vi "Define_KNRm.vi"() -> (0 "error out":errorcluster, 3 "KNR out":T1)   [LabVIEW 2013]
uses:
  <userlib>/KNR OS 3.0 LabVIEW Toolkit/Type Definition/KNR3 Reference.ctl
  <userlib>/_FPGA Interface Advanced Tools/FPGA Interface Base/FPGA Interface Base.lvclass
  <userlib>/KNR OS 3.0 LabVIEW Toolkit/Type Definition/Resource.ctl
  <userlib>/KNR OS 3.0 LabVIEW Toolkit/Type Definition/DC Motor Port.ctl
  <userlib>/KNR OS 3.0 LabVIEW Toolkit/Type Definition/RC Servo Port.ctl
  Global_KNRm.vi
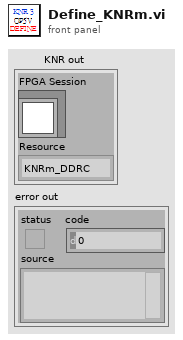
[diagram p1: front panel]
types:
  T1 = typedef "KNR3 Reference.ctl" = cluster{"FPGA Session":refnum<class "FPGA Interface Base.lvclass">, "Resource":T2}
  T2 = typedef "Resource.ctl" = enum16{"KNRm_DDRC", "KNRm_DDDD", "KNRm_DDDR", "KNRm_DDDC", "KNR"}
  T3 = typedef "DC Motor Port.ctl" = u16
  T4 = typedef "RC Servo Port.ctl" = u16
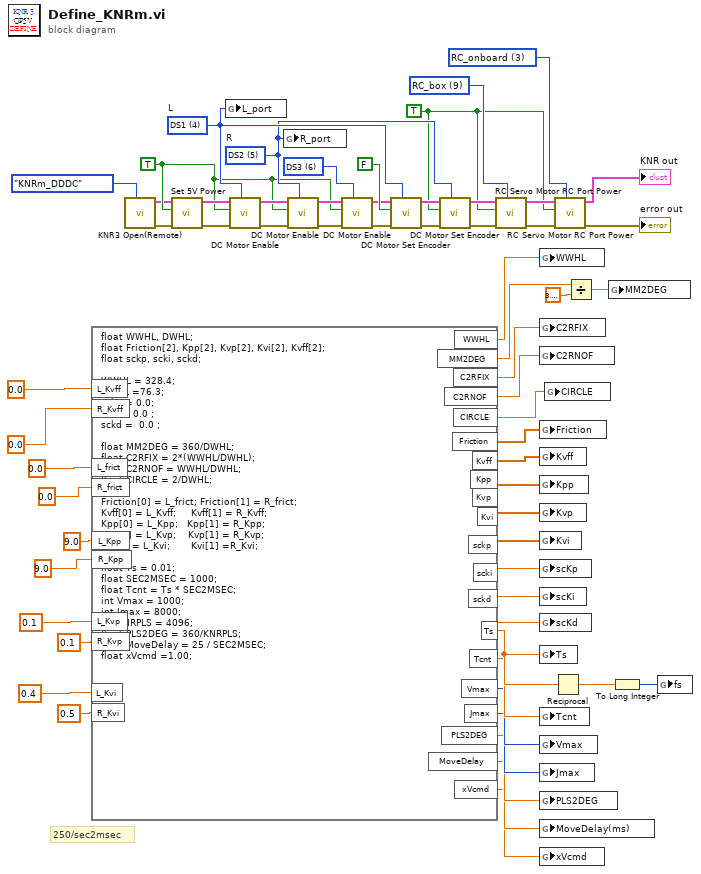
[diagram p0: block diagram]
diagram:
  w23 = T3 6 items=["DS1"=4, "DS2"=5, "DS3"=6, "DS4"=7] ("Port (DS1)")
  w28 = T4 3 items=["RC_onboard"=3, "RC_box"=9] ("Port (RC_onboard)")
  w32 = T4 9 items=["RC_onboard"=3, "RC_box"=9] ("Port (RC_onboard)")
  w56 = T3 5 items=["DS1"=4, "DS2"=5, "DS3"=6, "DS4"=7]  # R
  w57 = T3 4 items=["DS1"=4, "DS2"=5, "DS3"=6, "DS4"=7]  # L
  w29 = TRUE ("Reverse?(F)")
  w15 = TRUE ("Enable Motor(F)")
  # "250/sec2msec"
  n1 = formula code="float WWHL, DWHL;\nfloat Friction[2], Kpp[2], Kvp[2], Kvi[2], Kvff[2];\nfloat sckp, scki, sckd;\n\nWWHL = 328.4;\nDWHL =76.3;\nsckp = 0.0;\nscki = 0.0 ;\nsckd =  0.0 ;\n\nfloat MM2DEG = 360/DWHL;\nfloat C2RFIX = 2*(WWHL/DWHL);\nfloat C2RNOF = WWHL/DWHL;\nfloat CIRCLE = 2/DWHL;\n\nFriction[0] = L_frict; Friction[1] = R_frict;\nKvff[0] = L_Kvff;     Kvff[1] = R_Kvff;\nKpp[0] = L_Kpp;   Kpp[1] = R_Kpp;\nKvp[0] = L_Kvp;    Kvp[1] = R_Kvp;\nKvi[0] = L_Kvi;       Kvi[1] =R_Kvi;\n\nfloat Ts = 0.01;\nfloat SEC2MSEC = 1000;\nfloat Tcnt = Ts * SEC2MSEC;\nint Vmax = 1000;\nint Jmax = 8000;\nint KNRPLS = 4096;\nfloat PLS2DEG = 360/KNRPLS;\nfloat MoveDelay = 25 / SEC2MSEC;\nfloat xVcmd =1.00;"("L_Kvff"=0.0 ("input variable"), "R_Kvff"=0.0 ("input variable"), "L_frict"=0.0 ("input variable"), "R_frict"=0.0 ("input variable"), "L_Kpp"=9.0 ("input variable"), "R_Kpp"=9.0 ("input variable"), "L_Kvp"=0.1 ("input variable"), "R_Kvp"=0.1 ("input variable"), "L_Kvi"=0.4 ("input variable"), "R_Kvi"=0.5 ("input variable")) -> ("MM2DEG"=w20:dbl, "C2RFIX"=w52:dbl, "C2RNOF"=w51:dbl, "Friction"=w50:dbl[], "Kvff"=w49:dbl[], "Kpp"=w48:dbl[], "Kvp"=w47:dbl[], "Kvi"=w46:dbl[], "sckp"=w45:dbl, "scki"=w44:dbl, "sckd"=w43:dbl, "Ts"=w40:dbl, "Tcnt"=w39:dbl, "Vmax"=w38:i32, "Jmax"=w37:i32, "PLS2DEG"=w36:dbl, "WWHL"=w22:dbl, "MoveDelay"=w18:dbl, "xVcmd"=w14:dbl, "CIRCLE"=w1:dbl)
  n2 = call <userlib>:"KNR3 Open(Remote).vi"("Resource"=Resource."KNRm_DDDC") -> ("error out"=w12:errorcluster, "KNR out"=w13:T1)  [unwired: 9 in]
  n3 = call <userlib>:"Set 5V Power.vi"("error in (no error)"=w12, "5V Power(T)"=w15, "KNR in"=w13) -> ("error out"=w17:errorcluster, "KNR out"=w16:T1)  [unwired: 7 in]
  n4 = global write "Global_KNRm.vi" "L_port"(w57) -> ()
  n5 = call <userlib>:"DC Motor Enable.vi"("Port (DS1)"=w57, "error in (no error)"=w17, "Enable Motor(F)"=w15, "KNR in"=w16) -> ("error out"=w60:errorcluster, "KNR out"=w61:T1)  [unwired: 6 in]
  n6 = global write "Global_KNRm.vi" "R_port"(w56) -> ()
  n7 = call <userlib>:"DC Motor Enable.vi"("Port (DS1)"=w56, "error in (no error)"=w60, "Enable Motor(F)"=w15, "KNR in"=w61) -> ("error out"=w26:errorcluster, "KNR out"=w27:T1)  [unwired: 6 in]
  n8 = call <userlib>:"DC Motor Enable.vi"("Port (DS1)"=w23, "error in (no error)"=w26, "Enable Motor(F)"=w15, "KNR in"=w27) -> ("error out"=w25:errorcluster, "KNR out"=w24:T1)  [unwired: 6 in]
  n9 = call <userlib>:"DC Motor Set Encoder.vi"("Port (DS1)"=w57, "error in (no error)"=w25, "Reverse?(F)"=FALSE, "KNR in"=w24) -> ("error out"=w58:errorcluster, "KNR out"=w59:T1)  [unwired: 6 in]
  n10 = call <userlib>:"DC Motor Set Encoder.vi"("Port (DS1)"=w56, "error in (no error)"=w58, "Reverse?(F)"=w29, "KNR in"=w59) -> ("error out"=w33:errorcluster, "KNR out"=w34:T1)  [unwired: 6 in]
  n11 = call <userlib>:"RC Servo Motor RC Port Power.vi"("Port (RC_onboard)"=w32, "error in (no error)"=w33, "RC Power(F)"=w29, "KNR in"=w34) -> ("error out"=w30:errorcluster, "KNR out"=w31:T1)  [unwired: 6 in]
  n12 = global write "Global_KNRm.vi" "WWHL"(w22) -> ()
  n13 = global write "Global_KNRm.vi" "C2RFIX"(w52) -> ()
  n14 = global write "Global_KNRm.vi" "C2RNOF"(w51) -> ()
  n15 = global write "Global_KNRm.vi" "Friction"(w50) -> ()
  n16 = global write "Global_KNRm.vi" "Kvff"(w49) -> ()
  n17 = global write "Global_KNRm.vi" "Kpp"(w48) -> ()
  n18 = global write "Global_KNRm.vi" "Kvp"(w47) -> ()
  n19 = global write "Global_KNRm.vi" "Kvi"(w46) -> ()
  n20 = global write "Global_KNRm.vi" "scKp"(w45) -> ()
  n21 = global write "Global_KNRm.vi" "scKi"(w44) -> ()
  n22 = global write "Global_KNRm.vi" "scKd"(w43) -> ()
  n23 = global write "Global_KNRm.vi" "Ts"(w40) -> ()
  n24 = global write "Global_KNRm.vi" "Tcnt"(w39) -> ()
  n25 = global write "Global_KNRm.vi" "Vmax"(w38) -> ()
  n26 = global write "Global_KNRm.vi" "Jmax"(w37) -> ()
  n27 = global write "Global_KNRm.vi" "PLS2DEG"(w36) -> ()
  n28 = global write "Global_KNRm.vi" "MoveDelay(ms)"(w18) -> ()
  n29 = global write "Global_KNRm.vi" "xVcmd"(w14) -> ()
  n30 = global write "Global_KNRm.vi" "CIRCLE"(w1) -> ()
  n31 = Reciprocal(x=w40) -> (1/x=w42:dbl)
  n32 = call <userlib>:"RC Servo Motor RC Port Power.vi"("Port (RC_onboard)"=w28, "error in (no error)"=w30, "RC Power(F)"=w29, "KNR in"=w31) -> ("error out"=→"error out":errorcluster, "KNR out"=→"KNR out":T1)  [unwired: 6 in]
  n33 = Divide(x=w20, y=3.141592653589793) -> (x/y=w19:dbl)
  n34 = global write "Global_KNRm.vi" "MM2DEG"(w19) -> ()
  n35 = To Long Integer(number=w42) -> (32bit integer=w41:i32)
  n36 = global write "Global_KNRm.vi" "fs"(w41) -> ()
